vi "GT Add Task.vi"(7 "pTaskIndex":i16, 8 "error in (no error)":errorcluster caption="错误输入（无错误）", 9 "pTaskData":cluster{"mask":i16, "option":i16}, 10 "taskType":i16, 11 "cardNum":i16) -> (0 "error out":errorcluster caption="错误输出", 1 "pTaskData 2":cluster{"mask":i16, "option":i16}, 3 "cardNum":i16, 5 "pTaskIndex out":i16)   [LabVIEW 2020, in "gts1.lvlib"]
doc: "GT_API GT_AddTask(short cardNum,short taskType,void *pTaskData,short *pTaskIndex);"
uses:
  gts1.lvlib
  dll/32bit/multi_card/gts.dll
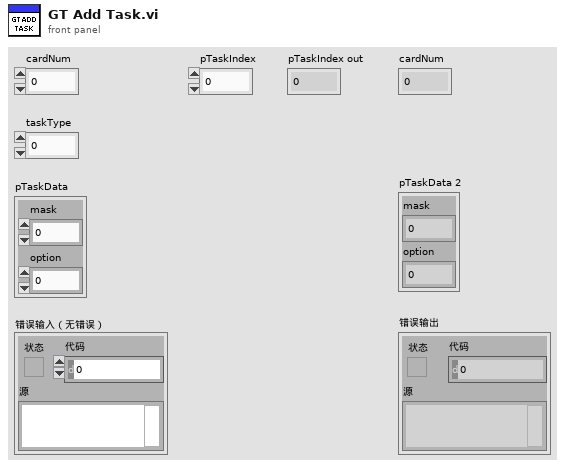
[diagram p1: front panel]
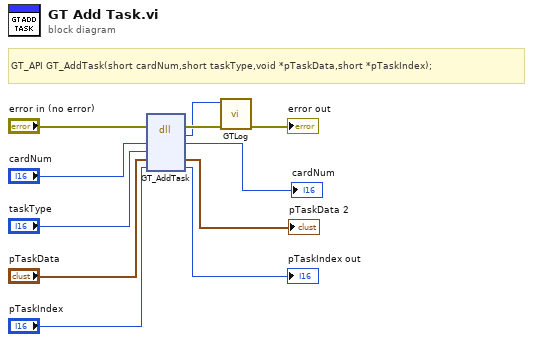
[diagram p0: block diagram]
diagram:
  # "GT_API GT_AddTask(short cardNum,short taskType,void *pTaskData,short *pTaskIndex);"
  n1 = dll-call lib="D:/Git/GoogolCard/dll/32bit/multi_card/gts.dll" fn="GT_AddTask"(error in="error in (no error)", "cardNum"="cardNum", "taskType"="taskType", "pTaskData"="pTaskData", "pTaskIndex"="pTaskIndex") -> (error out=w5:errorcluster, "返回类型"=w2:i16, "cardNum"=→"cardNum":i16, "pTaskData"=→"pTaskData 2":cluster{"mask":i16, "option":i16}, "pTaskIndex"=→"pTaskIndex out":i16)  [unwired: 3 in, 1 out]
  n2 = call "GTLog.vi"("error in (no error)"=w5, "Numeric"=w2) -> ("error out"=→"error out":errorcluster)  [unwired: 9 in]
